vi "AlphaBetaToDQ_src.vi"(0 "alpha":sgl format="%#_32g", 5 "beta":sgl format="%#_32g", 7 "theta":sgl) -> (4 "direct":sgl, 6 "quadrature":sgl)   [LabVIEW 2015]
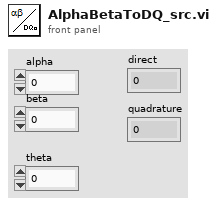
[diagram p1: front panel]
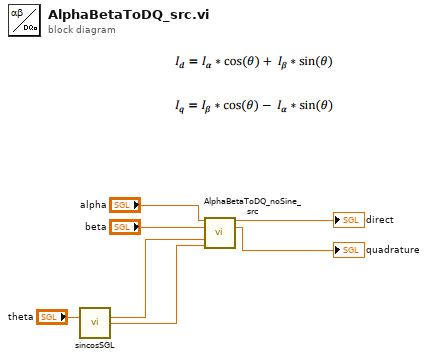
[diagram p0: block diagram]
diagram:
  n1 = call "sincosSGL.vi"("x"="theta") -> ("sinx"=w4:sgl, "cosx"=w3:sgl)  [unwired: 13 in]
  n2 = call "AlphaBetaToDQ_noSine_src.vi"("alpha"="alpha", "beta"="beta", "sinx"=w4, "cosx"=w3) -> ("direct"=→"direct":sgl, "quadrature"=→"quadrature":sgl)  [unwired: 10 in]
